vi "Teleop.vi"(10 "Match Info":T1={"Autonomous Elapsed Seconds"=0.0, "TeleOp Elapsed Seconds"=0.0, "Disabled Elapsed Seconds"=0.0, "Visited Autonomous"=FALSE, "Visited TeleOp"=FALSE, "Visited Disabled"=FALSE, "Autonomous Settings"={"Autonomous Style"=enum."Independent", "VI Refnum"=refnum}}, 11 "Call Context":T2) -> ()   [LabVIEW 2020]
doc: "This VI is called for each TeleOp packet received from the DS where the robot is not disabled. It is often used to read from the joysticks and update I/O or to update setpoints for timed control loops. It should complete and return within 20 milliseconds or it may miss DS packets."
uses:
  <vilib>/Rock Robotics/WPI/DriverStation/WPI_DriverStationDerivedRobotMode.ctl
  <vilib>/Rock Robotics/WPI/DriverStation/WPI_DriverStationMatch Info.ctl
  <vilib>/Rock Robotics/WPI/Joystick/XBox Axes Indexer.ctl
  <vilib>/Rock Robotics/WPI/ThirdParty/Phoenix-LabVIEW/Motor Controller/Controls/CTRE_Phoenix_MotorControl_ControlMode.ctl
  <vilib>/Rock Robotics/WPI/Utilities/WPI_GetSetVariantRefNum.vi
  <vilib>/Rock Robotics/Network Tables/NT Write Numeric Array.vi
  <vilib>/Rock Robotics/Network Tables/NT Read Boolean.vi
  <vilib>/Rock Robotics/WPI/ThirdParty/Phoenix-LabVIEW/Motor Controller/Get/CTRE_Phoenix_MotorController_GetSelectedSensorData.vi
  <vilib>/Rock Robotics/Network Tables/NT Write Boolean Array.vi
  <vilib>/Rock Robotics/Network Tables/NT Read Number.vi
panel:
  out "Voltage":dbl
  out "Sample Slider 0":dbl(slide) scale=0.0..5.0
  out "Sample Boolean 1":bool
  out "Sample Boolean 0":bool
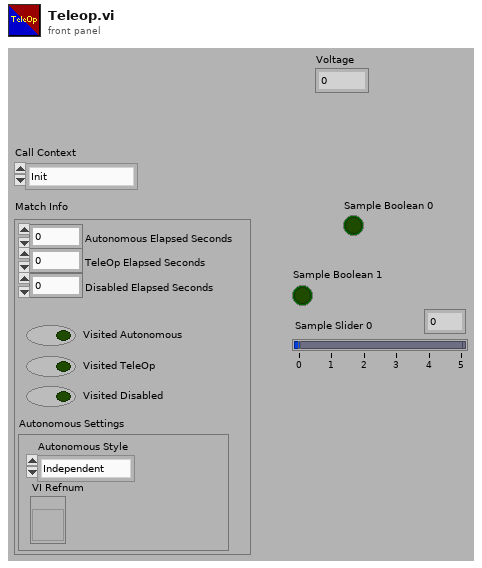
[diagram p1: front panel]
types:
  T1 = typedef "WPI_DriverStationMatch Info.ctl" = cluster{"Autonomous Elapsed Seconds":dbl, "TeleOp Elapsed Seconds":dbl, "Disabled Elapsed Seconds":dbl, "Visited Autonomous":bool, "Visited TeleOp":bool, "Visited Disabled":bool, "Autonomous Settings":cluster{"Autonomous Style":enum16{"Iterative", "Independent"}, "VI Refnum":refnum<vi>}}
  T2 = typedef "WPI_DriverStationDerivedRobotMode.ctl" = enum16{"Init", "Execute", "Stop"}
  T3 = typedef "CTRE_Phoenix_MotorControl_ControlMode.ctl" = u16
  T4 = typedef "XBox Axes Indexer.ctl" = enum16{"Left X", "Left Y", "Left Trigger", "Right Trigger", "Right X", "Right Y"}
  T5 = typedef "WPI_AnalogChannelDevRef.ctl" = cluster{"DevStatus":errorcluster, "Analog Channel":T6}
  T6 = typedef "FPGA_AIChannel.ctl" = enum8{"AI 0", "AI 1", "AI 2", "AI 3", "AI MXP 0", "AI MXP 1", "AI MXP 2", "AI MXP 3", "Invalid"}
  T7 = typedef "WPI_RobotDriveDevRef.ctl" = cluster{"DevStatus":errorcluster, "Motors[]":T8[], "Square Inputs":bool, "Max Output":dbl}
  T8 = typedef "WPI_MotorControlDeviceRef.ctl" = cluster{"DeviceStatus":errorcluster, "Type":T9, "PWM":cluster{"PWM Channel":T10, "DeadBand":T11}, "CAN":cluster{"Device Number":u8, "SetOutput VI Ref":variant, "GetOutput VI Ref":variant, "Enable VI Ref":variant, "Disable VI Ref":variant, "Data":variant}, "Invert":bool, "DIO PWM":cluster{"PWM \"Enable\" Channel":T10, "DIOChannel":T12, "PWM Rate":dbl}}
  T9 = typedef "WPI_MotorControlType.ctl" = enum16{"PWM", "CAN", "DIO PWM"}
  T10 = typedef "FPGA_DIOPWMChannel.ctl" = enum8{"PWM 0", "PWM 1", "PWM 2", "PWM 3", "PWM 4", "PWM 5", "PWM 6", "PWM 7", "PWM 8", "PWM 9", "PWM MXP 0", "PWM MXP 1", "PWM MXP 2", "PWM MXP 3", "PWM MXP 4", "PWM MXP 5", "PWM MXP 6", "PWM MXP 7", "PWM MXP 8", "PWM MXP 9", "Invalid"}
  T11 = typedef "WPI_PWMDeadband.ctl" = cluster{"Name":string, "maxPositivePwm":i32, "minPositivePwm":i32, "centerPwm":i32, "maxNegativePwm":i32, "minNegativePwm":i32, "angularRange":u16}
  T12 = typedef "FPGA_DIOChannel.ctl" = enum8{"DIO 0", "DIO 1", "DIO 2", "DIO 3", "DIO 4", "DIO 5", "DIO 6", "DIO 7", "DIO 8", "DIO 9", "DIO MXP 0", "DIO MXP 1", "DIO MXP 2", "DIO MXP 3", "DIO MXP 4", "DIO MXP 5", "DIO MXP 6", "DIO MXP 7", "DIO MXP 8", "DIO MXP 9", "DIO MXP 10", "DIO MXP 11", "DIO MXP 12", "DIO MXP 13", "DIO MXP 14", "DIO MXP 15", "SPI Port CS1", "SPI Port CS2", "SPI Port CS3", "SPI Port MISO", "SPI Port MOSI", "Invalid"}
  T13 = typedef "WPI_JoystickDevRef.ctl" = cluster{"Device":T14}
  T14 = typedef "WPI_JoystickDeviceEnum.ctl" = enum16{"USB 0", "USB 1", "USB 2", "USB 3", "USB 4", "USB 5"}
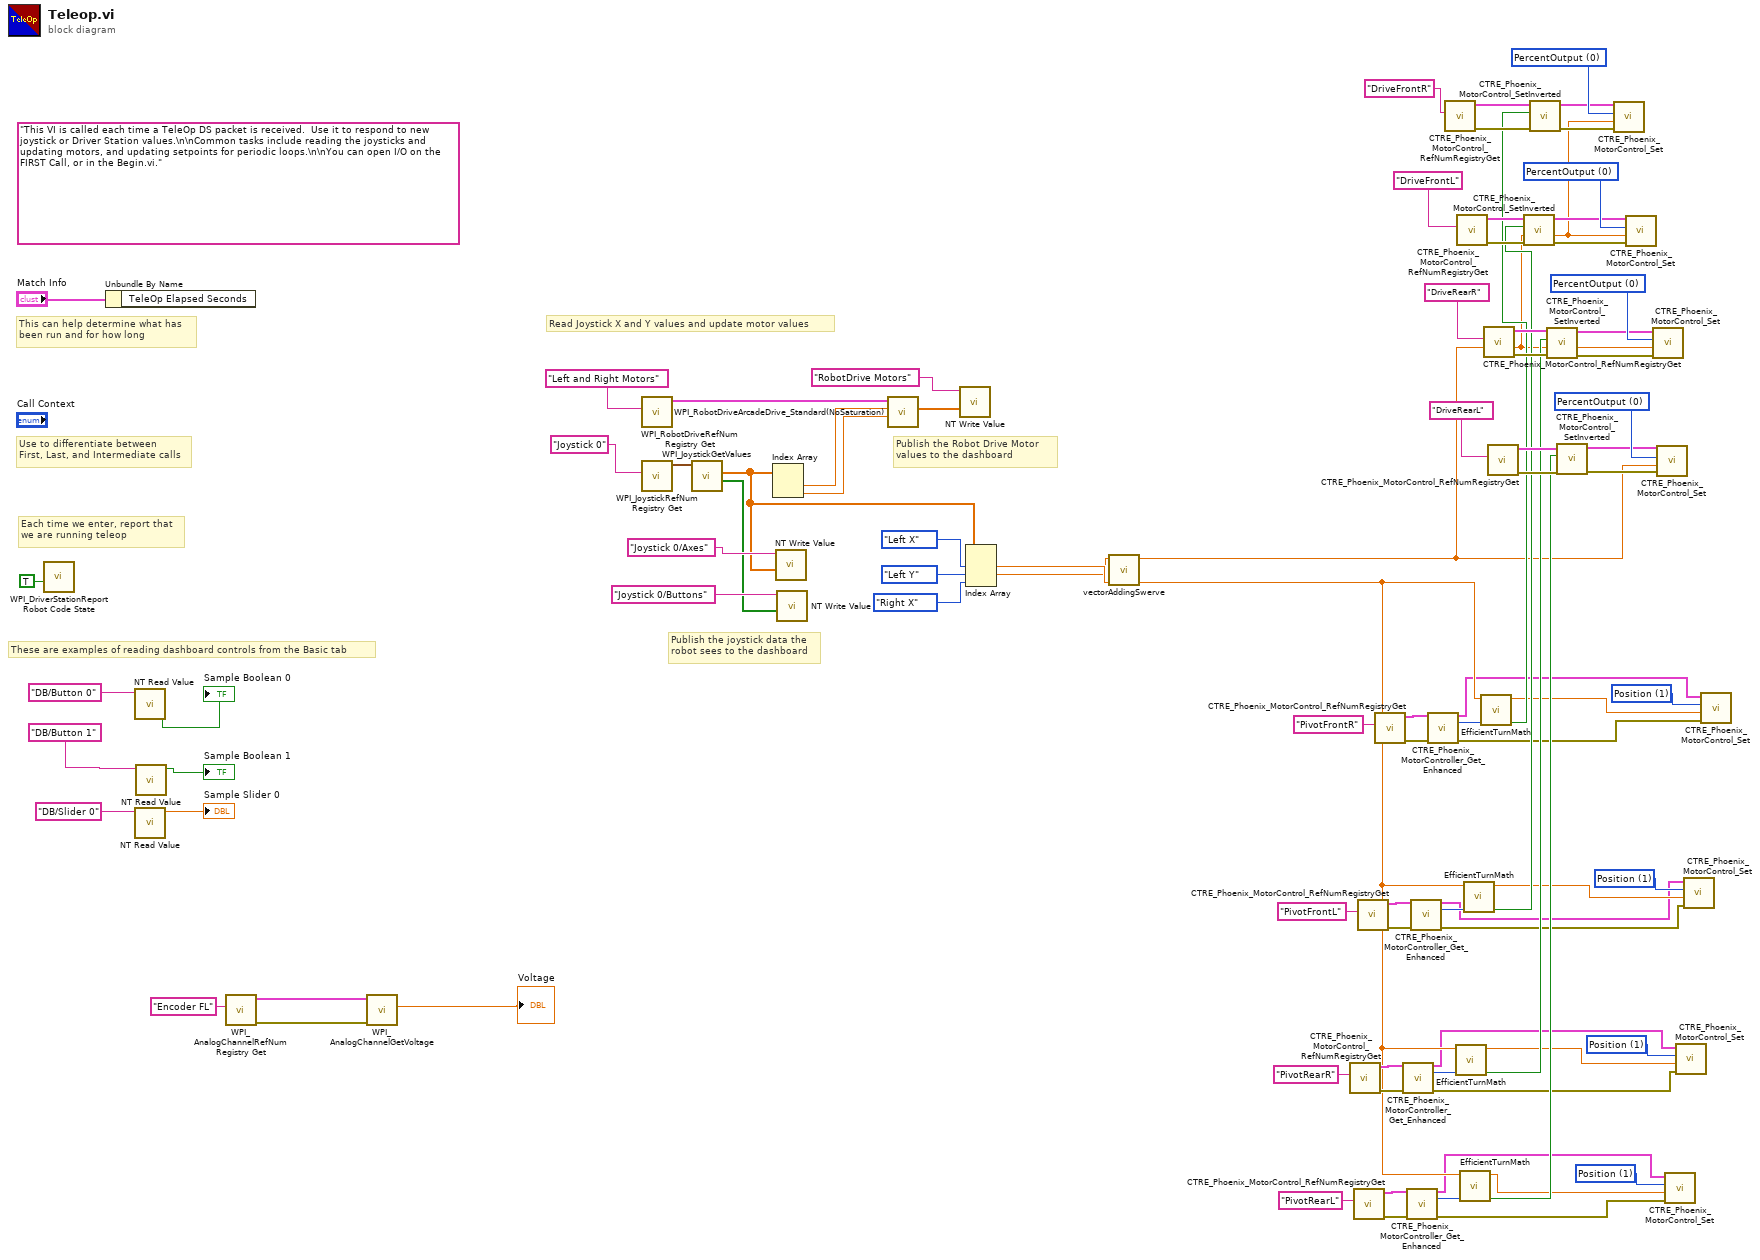
[diagram p0: block diagram]
diagram:
  w12 = T3 1 items=["PercentOutput"=0, "Position"=1, "Velocity"=2, "Current"=3, "Follower"=5, "MotionProfile"=6, "MotionMagic"=7, "MotionProfileArc"=10, "Disabled"=15] ("Control Mode")
  w13 = T3 1 items=["PercentOutput"=0, "Position"=1, "Velocity"=2, "Current"=3, "Follower"=5, "MotionProfile"=6, "MotionMagic"=7, "MotionProfileArc"=10, "Disabled"=15] ("Control Mode")
  w14 = T3 1 items=["PercentOutput"=0, "Position"=1, "Velocity"=2, "Current"=3, "Follower"=5, "MotionProfile"=6, "MotionMagic"=7, "MotionProfileArc"=10, "Disabled"=15] ("Control Mode")
  w16 = T3 1 items=["PercentOutput"=0, "Position"=1, "Velocity"=2, "Current"=3, "Follower"=5, "MotionProfile"=6, "MotionMagic"=7, "MotionProfileArc"=10, "Disabled"=15] ("Control Mode")
  w61 = T3 0 items=["PercentOutput"=0, "Position"=1, "Velocity"=2, "Current"=3, "Follower"=5, "MotionProfile"=6, "MotionMagic"=7, "MotionProfileArc"=10, "Disabled"=15] ("Control Mode")
  w62 = T3 0 items=["PercentOutput"=0, "Position"=1, "Velocity"=2, "Current"=3, "Follower"=5, "MotionProfile"=6, "MotionMagic"=7, "MotionProfileArc"=10, "Disabled"=15] ("Control Mode")
  w65 = T3 0 items=["PercentOutput"=0, "Position"=1, "Velocity"=2, "Current"=3, "Follower"=5, "MotionProfile"=6, "MotionMagic"=7, "MotionProfileArc"=10, "Disabled"=15] ("Control Mode")
  w66 = T3 0 items=["PercentOutput"=0, "Position"=1, "Velocity"=2, "Current"=3, "Follower"=5, "MotionProfile"=6, "MotionMagic"=7, "MotionProfileArc"=10, "Disabled"=15] ("Control Mode")
  (unwired) "This VI is called each time a TeleOp DS packet is received.  Use it to respond to new joystick or Driver Station values.\n\nCommon tasks include reading the joysticks and updating motors, and updating setpoints for periodic loops.\n\nYou can open I/O on the FIRST Call, or in the Begin.vi."
  # "These are examples of reading dashboard controls from the Basic tab"
  # "Publish the Robot Drive Motor\nvalues to the dashboard"
  # "Publish the joystick data the\nrobot sees to the dashboard"
  # "Each time we enter, report that\nwe are running teleop"
  # "Use to differentiate between\nFirst, Last, and Intermediate calls"
  # "This can help determine what has\nbeen run and for how long"
  # "Read Joystick X and Y values and update motor values"
  n1 = call <vilib>:"WPI_DriverStationReport Robot Code State.vi"("TeleOp"=TRUE ("Autonomous")) -> ()  [unwired: 10 in, 1 out]
  n2 = Unbundle By Name("Match Info") -> ()  [unwired: 1 out]
  n3 = call-poly <vilib>:"NT Read Value.vi"("Name"="DB/Button 0" ("refnum name")) -> ("Boolean"=→"Sample Boolean 0":bool)  [unwired: 9 in, 1 out]
  n4 = call-poly <vilib>:"NT Read Value.vi"("Name"="DB/Slider 0" ("refnum name")) -> ("Numeric"=→"Sample Slider 0":dbl)  [unwired: 9 in, 1 out]
  n5 = call-poly <vilib>:"NT Read Value.vi"("Name"="DB/Button 1" ("refnum name")) -> ("Boolean"=→"Sample Boolean 1":bool)  [unwired: 9 in, 1 out]
  n6 = call <vilib>:"WPI_AnalogChannelRefNum Registry Get.vi"("refnum name"="Encoder FL") -> ("error out"=w22:errorcluster, "AIDeviceRef"=w23:T5)  [unwired: 9 in]
  n7 = call <vilib>:"WPI_AnalogChannelGetVoltage.vi"("error in (no error)"=w22, "AIDeviceRef"=w23) -> ("Voltage"=→"Voltage":dbl)  [unwired: 7 in, 2 out]
  n8 = call <vilib>:"WPI_RobotDriveRefNum Registry Get.vi"("refnum name"="Left and Right Motors") -> ("RobotDriveDevRef"=w89:T7)  [unwired: 1 in, 9 out]
  n9 = call <vilib>:"WPI_JoystickRefNum Registry Get.vi"("refnum name"="Joystick 0") -> ("JoystickDevRef"=w86:T13)  [unwired: 1 in, 9 out]
  n10 = call <vilib>:"WPI_JoystickGetValues.vi"("JoystickDevRef"=w86) -> ("Buttons"=w81:bool[], "Axes"=w72:dbl[])  [unwired: 6 in, 3 out]
  n11 = Index Array(array=w72) -> (element #1=w88:dbl, element #2=w84:dbl)  [unwired: 2 in]
  n12 = call-poly <vilib>:"NT Write Value.vi"("Numeric Array"=w72, "Name"="Joystick 0/Axes") -> ()  [unwired: 9 in, 1 out]
  n13 = call-poly <vilib>:"NT Write Value.vi"("Boolean Array"=w81, "Name"="Joystick 0/Buttons") -> ()  [unwired: 9 in, 1 out]
  n14 = call <vilib>:"WPI_RobotDriveArcadeDrive_Standard(NoSaturation).vi"("Y axis value"=w84, "X axis value"=w88, "RobotDriveDevRef"=w89) -> ("Motor Values"=w74:dbl[])  [unwired: 1 in, 7 out]
  n15 = call-poly <vilib>:"NT Write Value.vi"("Numeric Array"=w74, "Name"="RobotDrive Motors") -> ()  [unwired: 9 in, 1 out]
  n16 = Index Array(array=w72, index #1=XBox_Axes_Indexer."Left X" ("XBox Axes"), index #2=XBox_Axes_Indexer."Left Y" ("XBox Axes"), index #3=XBox_Axes_Indexer."Right X" ("XBox Axes")) -> (element #1=w20:dbl, element #2=w19:dbl)  [unwired: 1 out]
  n17 = call "vectorAddingSwerve.vi"("LeftX"=w20, "LeftY"=w19) -> ("FinalAngle"=w17:dbl, "FinalVelocity"=w18:dbl)  [unwired: 8 in]
  n18 = call <vilib>:"CTRE_Phoenix_MotorControl_RefNumRegistryGet.vi"("refnum name"="PivotRearR") -> ("error out"=w36:errorcluster, "PhoenixMotorControlDevRef"=w35:T8)  [unwired: 9 in]
  n19 = call <vilib>:"CTRE_Phoenix_MotorControl_RefNumRegistryGet.vi"("refnum name"="PivotRearL") -> ("error out"=w39:errorcluster, "PhoenixMotorControlDevRef"=w40:T8)  [unwired: 9 in]
  n20 = call <vilib>:"CTRE_Phoenix_MotorControl_RefNumRegistryGet.vi"("refnum name"="PivotFrontL") -> ("error out"=w42:errorcluster, "PhoenixMotorControlDevRef"=w43:T8)  [unwired: 9 in]
  n21 = call <vilib>:"CTRE_Phoenix_MotorControl_RefNumRegistryGet.vi"("refnum name"="PivotFrontR") -> ("error out"=w33:errorcluster, "PhoenixMotorControlDevRef"=w32:T8)  [unwired: 9 in]
  n22 = call-poly <vilib>:"CTRE_Phoenix_MotorController_Get_Enhanced.vi"("PhoenixMotorControlDevRef"=w35, "error in"=w36) -> ("PhoenixMotorControlDevRef"=w6:T8, "Position (Raw Sensor Units)"=w37:i32, "error out"=w4:errorcluster)  [unwired: 10 in, 1 out]
  n23 = call-poly <vilib>:"CTRE_Phoenix_MotorController_Get_Enhanced.vi"("PhoenixMotorControlDevRef"=w40, "error in"=w39) -> ("PhoenixMotorControlDevRef"=w5:T8, "Position (Raw Sensor Units)"=w38:i32, "error out"=w1:errorcluster)  [unwired: 10 in, 1 out]
  n24 = call-poly <vilib>:"CTRE_Phoenix_MotorController_Get_Enhanced.vi"("PhoenixMotorControlDevRef"=w43, "error in"=w42) -> ("PhoenixMotorControlDevRef"=w7:T8, "Position (Raw Sensor Units)"=w41:i32, "error out"=w3:errorcluster)  [unwired: 10 in, 1 out]
  n25 = call-poly <vilib>:"CTRE_Phoenix_MotorController_Get_Enhanced.vi"("PhoenixMotorControlDevRef"=w32, "error in"=w33) -> ("PhoenixMotorControlDevRef"=w8:T8, "Position (Raw Sensor Units)"=w34:i32, "error out"=w2:errorcluster)  [unwired: 10 in, 1 out]
  n26 = call <vilib>:"CTRE_Phoenix_MotorControl_RefNumRegistryGet.vi"("refnum name"="DriveFrontR") -> ("error out"=w45:errorcluster, "PhoenixMotorControlDevRef"=w47:T8)  [unwired: 9 in]
  n27 = call "EfficientTurnMath.vi"("current"=w37, "target"=w17) -> ("Invert"=w25:bool, "AngleToTurn"=w9:dbl)  [unwired: 8 in]
  n28 = call <vilib>:"CTRE_Phoenix_MotorControl_RefNumRegistryGet.vi"("refnum name"="DriveFrontL") -> ("error out"=w49:errorcluster, "PhoenixMotorControlDevRef"=w51:T8)  [unwired: 9 in]
  n29 = call "EfficientTurnMath.vi"("current"=w38, "target"=w17) -> ("Invert"=w26:bool, "AngleToTurn"=w15:dbl)  [unwired: 8 in]
  n30 = call "EfficientTurnMath.vi"("current"=w41, "target"=w17) -> ("Invert"=w27:bool, "AngleToTurn"=w10:dbl)  [unwired: 8 in]
  n31 = call "EfficientTurnMath.vi"("current"=w34, "target"=w17) -> ("Invert"=w24:bool, "AngleToTurn"=w11:dbl)  [unwired: 8 in]
  n32 = call <vilib>:"CTRE_Phoenix_MotorControl_RefNumRegistryGet.vi"("refnum name"="DriveRearR") -> ("error out"=w53:errorcluster, "PhoenixMotorControlDevRef"=w55:T8)  [unwired: 9 in]
  n33 = call <vilib>:"CTRE_Phoenix_MotorControl_RefNumRegistryGet.vi"("refnum name"="DriveRearL") -> ("error out"=w58:errorcluster, "PhoenixMotorControlDevRef"=w59:T8)  [unwired: 9 in]
  n34 = call <vilib>:"CTRE_Phoenix_MotorControl_SetInverted.vi"("error in (no error)"=w49, "Invert?"=w27, "PhoenixMotorControlDevRef"=w51) -> ("error out"=w48:errorcluster, "PhoenixMotorControlDevRef"=w50:T8)  [unwired: 7 in]
  n35 = call <vilib>:"CTRE_Phoenix_MotorControl_SetInverted.vi"("error in (no error)"=w45, "Invert?"=w24, "PhoenixMotorControlDevRef"=w47) -> ("error out"=w44:errorcluster, "PhoenixMotorControlDevRef"=w46:T8)  [unwired: 7 in]
  n36 = call <vilib>:"CTRE_Phoenix_MotorControl_SetInverted.vi"("error in (no error)"=w53, "Invert?"=w25, "PhoenixMotorControlDevRef"=w55) -> ("error out"=w52:errorcluster, "PhoenixMotorControlDevRef"=w54:T8)  [unwired: 7 in]
  n37 = call <vilib>:"CTRE_Phoenix_MotorControl_SetInverted.vi"("error in (no error)"=w58, "Invert?"=w26, "PhoenixMotorControlDevRef"=w59) -> ("error out"=w56:errorcluster, "PhoenixMotorControlDevRef"=w57:T8)  [unwired: 7 in]
  n38 = call <vilib>:"CTRE_Phoenix_MotorControl_Set.vi"("error in (no error)"=w44, "Output"=w18, "Control Mode"=w61, "PhoenixMotorControlDevRef"=w46) -> ()  [unwired: 6 in, 2 out]
  n39 = call <vilib>:"CTRE_Phoenix_MotorControl_Set.vi"("error in (no error)"=w48, "Output"=w18, "Control Mode"=w62, "PhoenixMotorControlDevRef"=w50) -> ()  [unwired: 6 in, 2 out]
  n40 = call <vilib>:"CTRE_Phoenix_MotorControl_Set.vi"("error in (no error)"=w52, "Output"=w18, "Control Mode"=w65, "PhoenixMotorControlDevRef"=w54) -> ()  [unwired: 6 in, 2 out]
  n41 = call <vilib>:"CTRE_Phoenix_MotorControl_Set.vi"("error in (no error)"=w56, "Output"=w18, "Control Mode"=w66, "PhoenixMotorControlDevRef"=w57) -> ()  [unwired: 6 in, 2 out]
  n42 = call <vilib>:"CTRE_Phoenix_MotorControl_Set.vi"("error in (no error)"=w1, "Output"=w15, "Control Mode"=w16, "PhoenixMotorControlDevRef"=w5) -> ()  [unwired: 6 in, 2 out]
  n43 = call <vilib>:"CTRE_Phoenix_MotorControl_Set.vi"("error in (no error)"=w4, "Output"=w9, "Control Mode"=w14, "PhoenixMotorControlDevRef"=w6) -> ()  [unwired: 6 in, 2 out]
  n44 = call <vilib>:"CTRE_Phoenix_MotorControl_Set.vi"("error in (no error)"=w3, "Output"=w10, "Control Mode"=w13, "PhoenixMotorControlDevRef"=w7) -> ()  [unwired: 6 in, 2 out]
  n45 = call <vilib>:"CTRE_Phoenix_MotorControl_Set.vi"("error in (no error)"=w2, "Output"=w11, "Control Mode"=w12, "PhoenixMotorControlDevRef"=w8) -> ()  [unwired: 6 in, 2 out]
